vi "create test channels.vi"() -> (0 "error out":errorcluster, 1 "Array":refnum<class "Modbus Module Channel.lvclass">[](array[class]), 2 "port (502)":u16, 3 "Modbus Slave configuration out":refnum<class "Modbus Slave configuration.lvclass">, 5 "names":string[](array[string]))   [LabVIEW 2013, in "Modbus Slave tests.lvlib"]
uses:
  Modbus Slave tests.lvlib
  module channel/Modbus Module Channel.lvclass
  configuration/Modbus Slave configuration.lvclass
  <vilib>/NI/Tag Bus Module Framework/channel/channel classification.ctl
  module channel/data bank type.ctl
  configuration/Modbus Slave configuration.lvclass/Modbus Slave configuration.ctl
  <vilib>/NI/Tag Bus/tag/tag descriptor.lvclass/tag descriptor.ctl
  <vilib>/NI/Tag Bus Module Framework/channel/TBM channel.lvclass/TBM channel.ctl
  module channel/Modbus Module Channel.lvclass/Modbus Module Channel.ctl
  <vilib>/NI/Tag Bus/tag/write tag name.vi
  <vilib>/NI/Tag Bus/tag/write data type.vi
  <vilib>/NI/Tag Bus Module Framework/channel/Write channel classification.vi
  module channel/Write modbus type.vi
  module channel/Write starting address.vi
  configuration/Write port (502).vi
  <vilib>/NI/Tag Bus Module Framework/channel/TBM channel.lvclass
  <vilib>/NI/Tag Bus Module Framework/root configuration/TBM configuration.lvclass
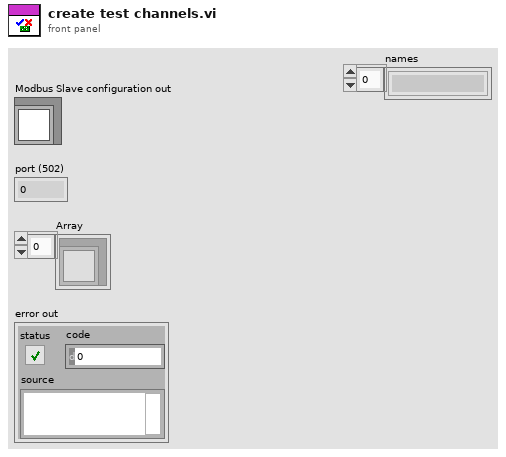
[diagram p1: front panel]
types:
  T1 = typedef "Modbus Module Channel.lvclass/data bank type.ctl" = enum16{"coils", "discrete inputs", "input registers", "holding registers"}
  T2 = typedef "TBM channel.lvclass/channel classification.ctl" = enum16{"input data", "output data", "processing parameter", "processing result"}
  T3 = typedef "tag bus.lvlib/tag descriptor.lvclass/Data Type.ctl" = enum16{"Double", "Single", "I64", "I32", "I16", "I8", "U64", "U32", "U16", "U8", "Boolean", "String", "Array of Double", "Array of Single", "Array of I64", "Array of I32", "Array of I16", "Array of I8", "Array of U64", "Array of U32", "Array of U16", "Array of U8", "Array of Boolean", "Array of String"}
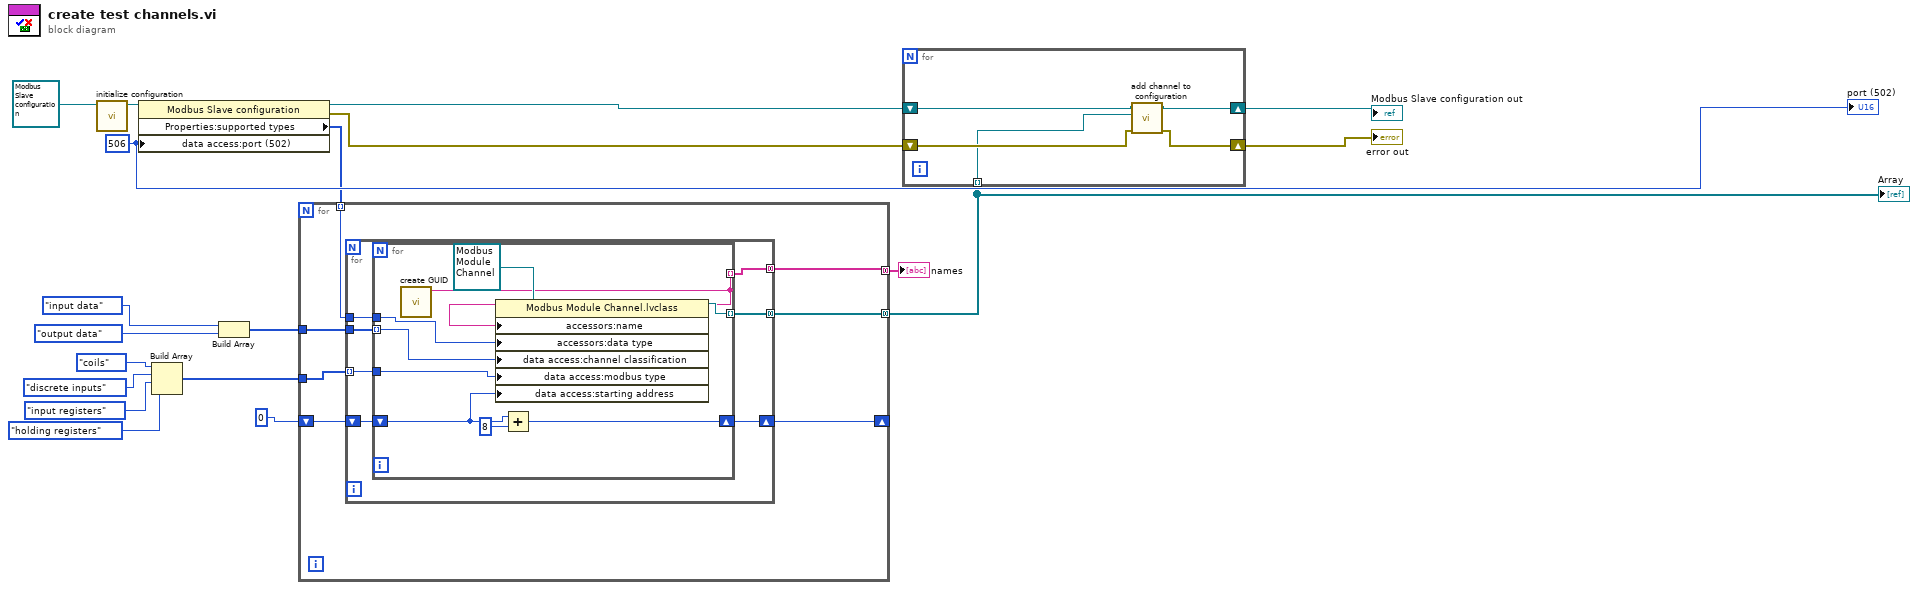
[diagram p0: block diagram]
diagram:
  w19 = u16 506 ("port (502)")
  n1 = call-dynamic "initialize configuration.vi"("configuration in"=refnum<class "Modbus Slave configuration.lvclass"> refnum ("tag bus configurable plugin module configuration")) -> ("configuration out"=w12:refnum<class "Modbus Slave configuration.lvclass">)  [unwired: 8 in, 2 out]
  n2 = property class="Modbus Slave configuration"(reference=w12, "data access:port (502)"=w19) -> (reference out=w6:refnum<class "Modbus Slave configuration.lvclass">, error out=w11:errorcluster, "Properties:supported types"=w5:T3[])  [unwired: 1 in]
  n3 = Build Array(data_bank_type."coils" ("modbus type"), data_bank_type."discrete inputs" ("modbus type"), data_bank_type."input registers" ("modbus type"), data_bank_type."holding registers" ("modbus type")) -> (w17:T1[])
  n4 = Build Array(channel_classification."input data" ("channel classification"), channel_classification."output data" ("channel classification")) -> (w4:T2[])
  n5 = for {
    tunnel: w4 -> [w26]
    tunnel: w5 -> [w25] mode=indexing
    tunnel: [w24] -> w9 mode=concatenating
    tunnel: w17 -> [w23]
    shift-right: [w22] -> _
    shift-left: u16 0 ("starting address") -> [w21]
    tunnel: [w20] -> w1 mode=concatenating
    n6 = for {
      tunnel: w26 -> [w33]
      tunnel: [w32] -> w24 mode=concatenating
      tunnel: w25 -> [w31]
      tunnel: w23 -> [w30] mode=indexing
      shift-right: [w29] -> w22
      shift-left: w21 -> [w28]
      tunnel: [w27] -> w20 mode=concatenating
      n7 = for {
        tunnel: w33 -> [w40] mode=indexing
        tunnel: [w41] -> w32 mode=indexing
        tunnel: w31 -> [w39]
        tunnel: w30 -> [w38]
        shift-right: [w37] -> w29
        shift-left: w28 -> [w36]
        tunnel: [w34] -> w27 mode=indexing
        n8 = call <vilib>:"create GUID.vi"() -> ("uuid"=w34:string)  [unwired: 11 in]
        n9 = property class="Modbus Module Channel.lvclass"(reference=refnum<class "Modbus Module Channel.lvclass"> refnum ("Modbus Module Channel.lvclass"), "accessors:name"=w34, "accessors:data type"=w39, "data access:channel classification"=w40, "data access:modbus type"=w38, "data access:starting address"=w36) -> (reference out=w41:refnum<class "Modbus Module Channel.lvclass">)  [unwired: 1 in, 1 out]
        n10 = Add(x=w36, y=u16 8) -> (x+y=w37:u16)
      }
    }
  }
  "Array" <- w9
  "names" <- w1
  n11 = for {
    tunnel: w9 -> [w45] mode=indexing
    shift-right: [w44] -> w8
    shift-left: w6 -> [w47]
    shift-right: [w43] -> w10
    shift-left: w11 -> [w46]
    n12 = call "add channel to configuration.vi"("error in"=w46, "Modbus Module Channel.lvclass"=w45, "Modbus Slave configuration in"=w47) -> ("error out"=w43:errorcluster, "Modbus Slave configuration out"=w44:refnum<class "Modbus Slave configuration.lvclass">)  [unwired: 7 in]
  }
  "error out" <- w10
  "Modbus Slave configuration out" <- w8
  "port (502)" <- w19
